vi "与非门逻辑实验.vi"() -> ()   [LabVIEW 2018]
panel:
  in  "结束":bool
  out "结果显示":bool
  in  "输入 2":bool
  in  "输入1":bool
  # "与或非逻辑实验"
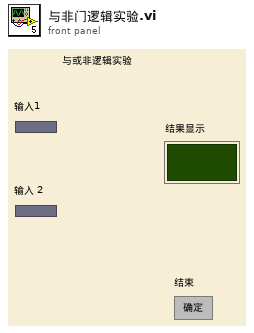
[diagram p1: front panel]
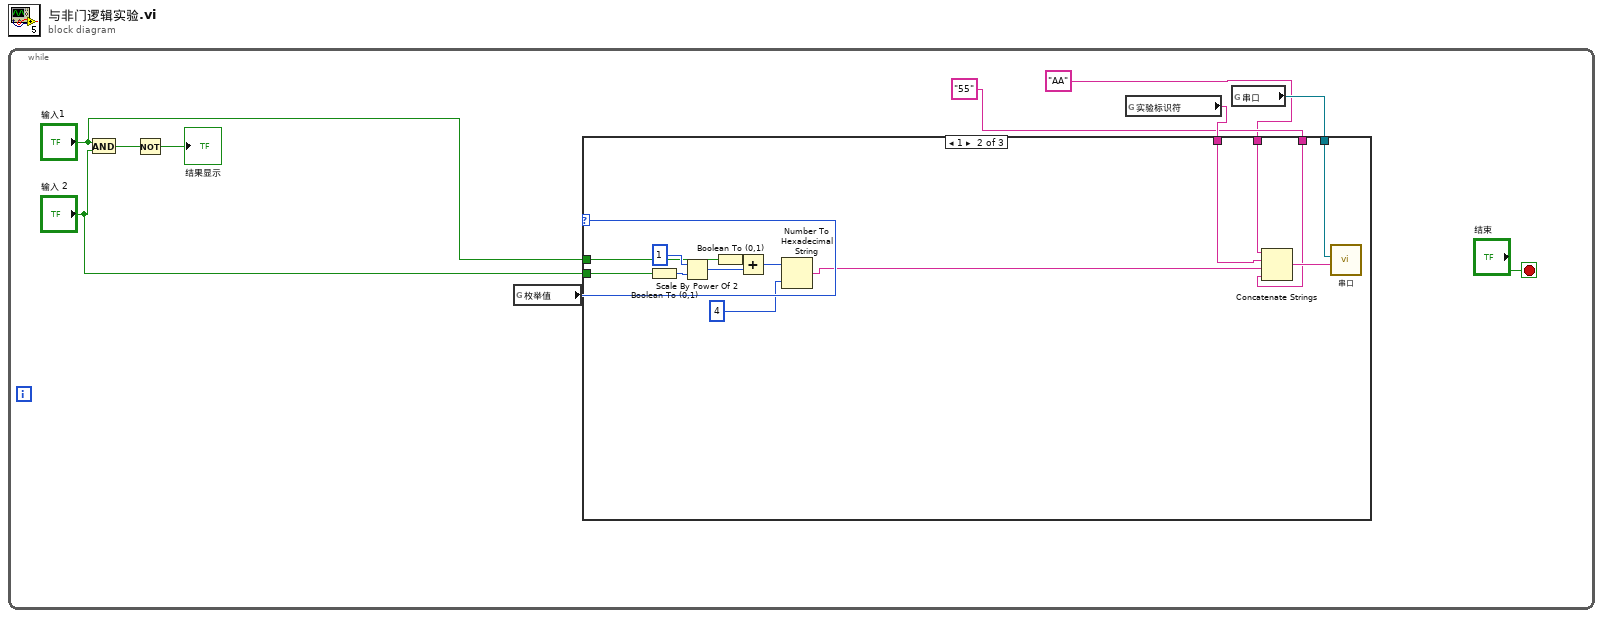
[diagram p0: block diagram]
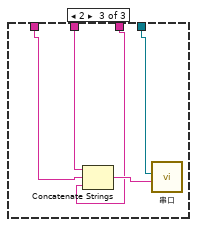
[diagram p3: hidden frame]
diagram:
  n1 = while {
    stop <- "结束" stop-if-true
    n2 = And(x="输入1", y="输入 2") -> (x .and. y?=w10:bool)
    n3 = Not(x=w10) -> (.not. x?=→"结果显示":bool)
    n4 = global read "全局变量.vi" "枚举值"() -> (w7:i8)
    n5 = global read "全局变量.vi" "实验标识符"() -> (w3:string)
    n6 = global read "全局变量.vi" "串口"() -> (w4:refnum<visa-resource-name>)
    n7 = case shown="1" w7 {
      tunnel: "输入 2" -> [_ w19 _]
      tunnel: "输入1" -> [_ w18 _]
      tunnel: w4 -> [_ w17 w27]
      tunnel: w3 -> [_ w16 w28]
      tunnel: "55" -> [_ w15 w25]
      tunnel: "AA" -> [_ w14 w26]
      frame 0, Default {
      }
      frame 1 {
        n8 = Boolean To (0,1)(Boolean=w19) -> (0, 1=w21:i16)
        n9 = Scale By Power Of 2(n=1, x=w21) -> (x*2^n=w22:i16)
        n10 = Boolean To (0,1)(Boolean=w18) -> (0, 1=w23:i16)
        n11 = Add(x=w23, y=w22) -> (x+y=w13:i16)
        n12 = Number To Hexadecimal String(1:4, 2:w13) -> (0:w11:string)
        n13 = Concatenate Strings(w14, w16, w11, w15) -> (w24:string)
        n14 = call "串口.vi"("字符串"=w24, "VISA resource name"=w17) -> ()  [unwired: 10 in]
      }
      frame 2 {
        n15 = Concatenate Strings(w26, w28, w25) -> (w29:string)
        n16 = call "串口.vi"("字符串"=w29, "VISA resource name"=w27) -> ()  [unwired: 10 in]
      }
    }
  }
